vi "查询前序设备.vi"(11 "PRODUCT_ID":string) -> (3 "前序工位":string[](array[string]))   [LabVIEW 2020]
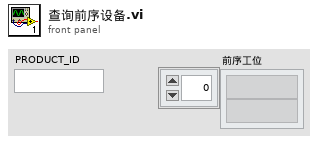
[diagram p1: front panel]
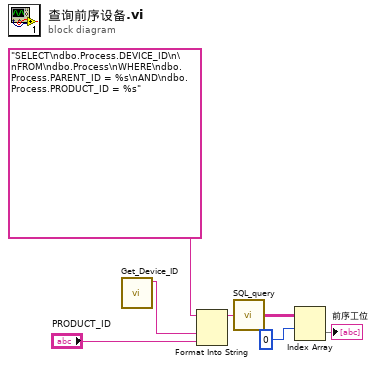
[diagram p0: block diagram]
diagram:
  n1 = call "Get_Device_ID.vi"() -> ("Device_ID"=w2:string)  [unwired: 10 in, 1 out]
  n2 = Format Into String(format string="SELECT\ndbo.Process.DEVICE_ID\n\nFROM\ndbo.Process\nWHERE\ndbo.Process.PARENT_ID = %s\nAND\ndbo.Process.PRODUCT_ID = %s" ("SQL query"), w2, "PRODUCT_ID") -> (resulting string=w6:string)  [unwired: 2 in, 1 out]
  n3 = call "SQL_query.vi"("SQL query"=w6) -> ("data"=w5:string[][])  [unwired: 2 in, 2 out]
  n4 = Index Array(array=w5, index (row)=0 ("禁用的索引 (列)")) -> (element=→"前序工位":string[])  [unwired: 1 in]
